vi "Crv_Info_Pan.vi"(8 "error in (no error)":errorcluster caption="entrée d'erreur (pas d'erreur)") -> (0 "error out":errorcluster caption="sortie d'erreur")   [LabVIEW 2019]
panel:
  out "EdPanelName":string="Scale & Offset"
  in  "Y Scale":dbl=60.0 min=0.1 step=0.1 format="%#.3f"
  in  "X Scale":dbl=60.0 min=0.1 step=0.1 format="%#.3f"
  in  "Y Offset":dbl caption="Offset" format="%.3f"
  in  "X Offset":dbl caption="Offset" format="%.3f"
  out "X Data Out":dbl[][](array[numeric])
  in  "XData":dbl[][](array[numeric])
  out "Y Data Out":dbl[][](array[numeric])
  in  "YData":dbl[][](array[numeric])
  in  "Apply_to":enum16{"X Data", "Y Data"}(ring) caption="Apply to:"
  in  "Quick Scale":dbl(slide) scale=0.0..6.0
  in  "Quick Offset":dbl(slide) scale=0.0..4.0
  in  "EditorProgQ":refnum<queue>
  in  "EditorProgQEvent":refnum<user-event>
  in  "Stop":bool
  in  "Offset":dbl format="%.3f"
  in  "Scale":dbl=60.0 format="%#.3f"
  out "Init Program":bool
  # "this MUST be present and labeled \"Stop\""
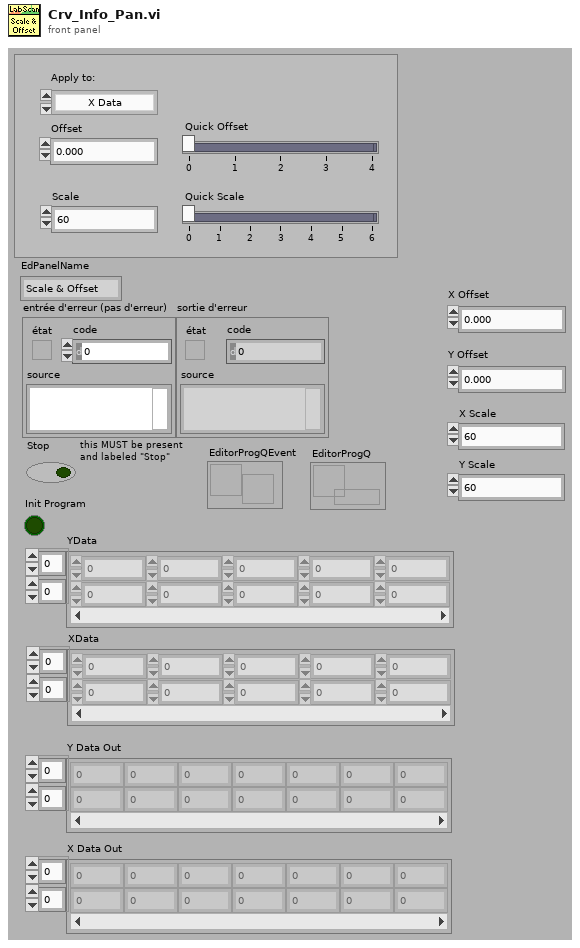
[diagram p1: front panel]
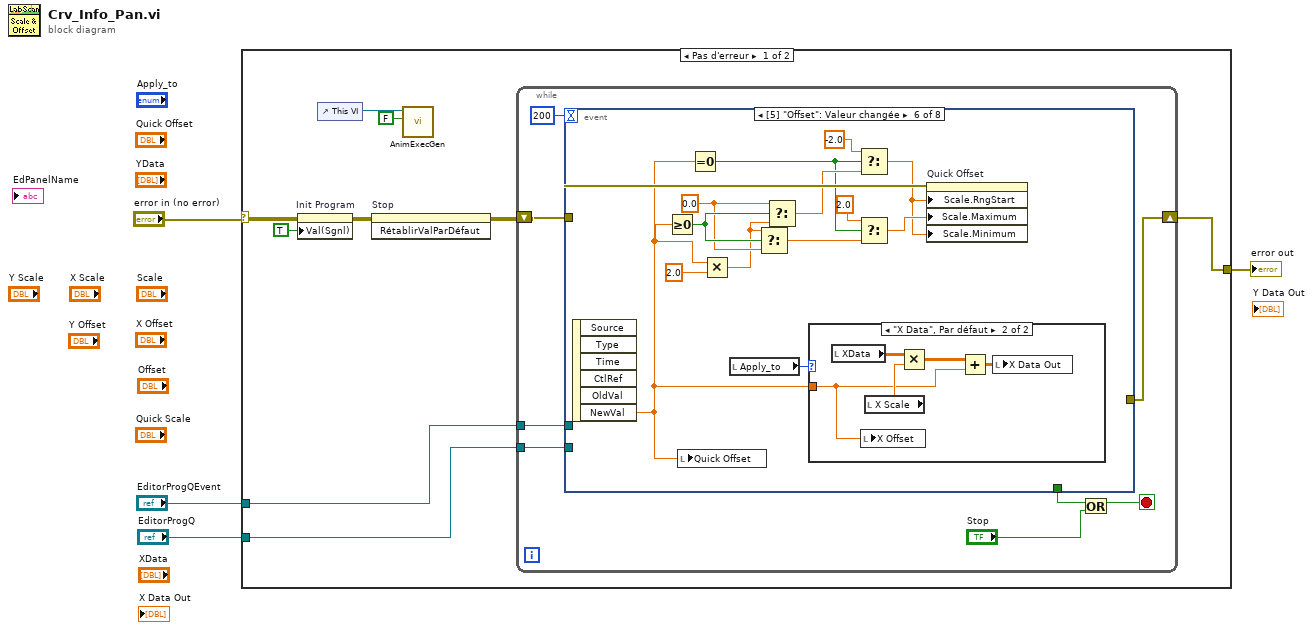
[diagram p0: block diagram]
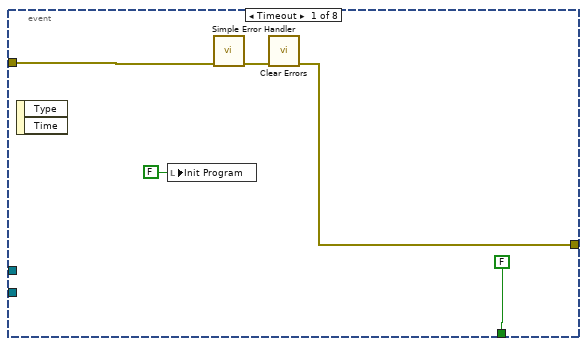
[diagram p2: hidden frame]
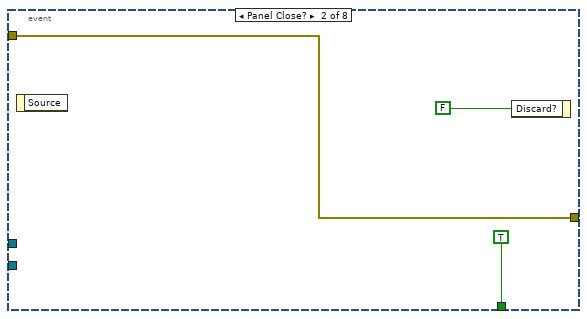
[diagram p3: hidden frame]
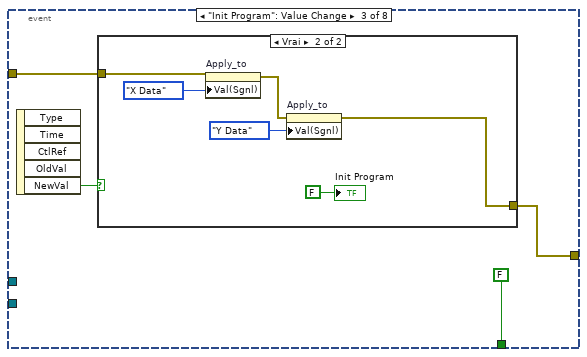
[diagram p4: hidden frame]
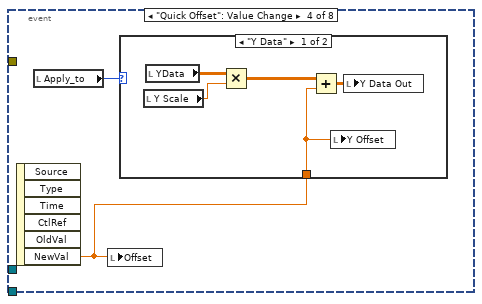
[diagram p6: hidden frame]
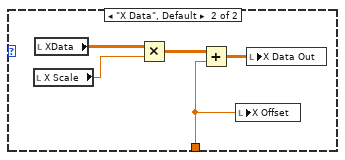
[diagram p7: hidden frame]
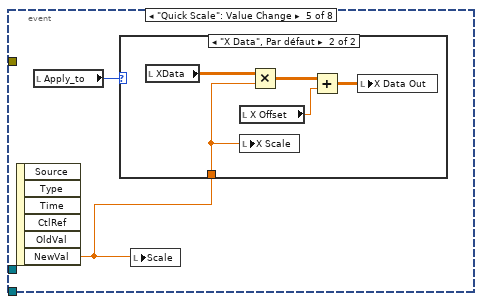
[diagram p8: hidden frame]
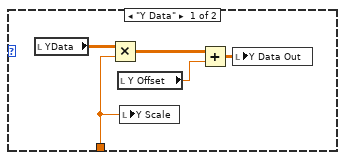
[diagram p9: hidden frame]
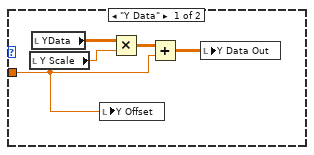
[diagram p10: hidden frame]
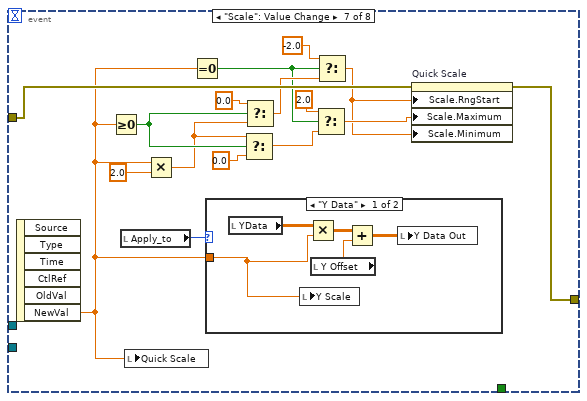
[diagram p11: hidden frame]
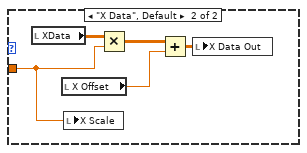
[diagram p12: hidden frame]
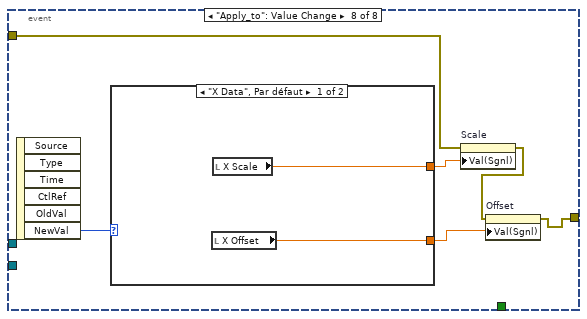
[diagram p13: hidden frame]
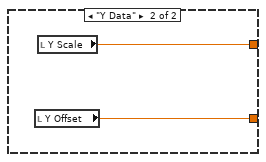
[diagram p14: hidden frame]
diagram:
  n1 = case shown="Pas d'erreur" "error in (no error)" {
    selector: "error in (no error)" -> [w11 w125]
    tunnel: [w13 w125] -> w3
    tunnel: "EditorProgQEvent" -> [w6 _]
    tunnel: "EditorProgQ" -> [w5 _]
    frame No Error {
      n2 = property on="Init Program" class="Bool (strict)"(error in=w11, "Val(Sgnl)"=TRUE ("Valeur (Signalisation)")) -> (error out=w10:errorcluster)  [unwired: 1 in, 1 out]
      n3 = control-ref of="This VI"() -> (w7:refnum<vi>)
      n4 = invoke on="Stop" class="Bool (strict)" method="RétablirValParDéfaut"(error in=w10) -> (error out=w9:errorcluster)  [unwired: 2 in, 2 out]
      n5 = call <userlib>:"AnimExecGen.vi"("Animer l'exécution ?"=FALSE, "ViRef"=w7) -> ()  [unwired: 9 in, 1 out]
      n6 = while {
        shift-right: [w19] -> w13
        shift-left: w9 -> [w20]
        tunnel: w6 -> [w15]
        tunnel: w5 -> [w14]
        stop <- w17 stop-if-true
        n7 = event shown="[5] \"Offset\": Valeur changée" {
          selector: _ -> [_ _ _ _ _ _ _ _]
          dyn-events: _ -> [_ _ _ _ _ _ _ _]
          timeout: 200 -> [_ _ _ _ _ _ _ _]
          tunnel: w20 -> [w25 w27 w32 _ _ w78 w104 w120]
          tunnel: [w23 w27 w31 _ _ _ w97 w115] -> w19
          tunnel: [FALSE TRUE FALSE _ _ _ _ _] -> w18
          tunnel: w15 -> [_ _ _ _ _ _ _ _]
          tunnel: w14 -> [_ _ _ _ _ _ _ _]
          event Timeout {
            n8 = event-data() -> ()  [unwired: 1 in, 2 out]
            n9 = local write "Init Program"(FALSE ("Init Program")) -> ()
            n10 = call <vilib>:"Simple Error Handler.vi"("error in (no error)"=w25) -> ("error out"=w24:errorcluster)  [unwired: 4 in, 4 out]
            n11 = call <vilib>:"Clear Errors.vi"("error in (no error)"=w24) -> ("error out"=w23:errorcluster)  [unwired: 5 in, 1 out]
          }
          event Panel Close? {
            n12 = event-data() -> ()  [unwired: 1 in, 1 out]
            n13 = event-data("Discard?"=FALSE ("Rejeter ?")) -> ()  [unwired: 1 in, 1 out]
          }
          event "Init Program": Value Change {
            n14 = event-data() -> ("NewVal"=w33:bool)  [unwired: 1 in, 4 out]
            n15 = case shown="Vrai" w33 {
              tunnel: w32 -> [w34 w37]
              tunnel: [w34 w39] -> w31
              frame False {
              }
              frame True {
                n16 = property on="Apply_to" class="Énum (strict)"(error in=w37, "Val(Sgnl)"=enum16{"X Data", "Y Data"}."X Data" ("Valeur (Signalisation)")) -> (error out=w36:errorcluster)  [unwired: 1 in, 1 out]
                n17 = property on="Apply_to" class="Énum (strict)"(error in=w36, "Val(Sgnl)"=enum16{"X Data", "Y Data"}."Y Data" ("Valeur (Signalisation)")) -> (error out=w39:errorcluster)  [unwired: 1 in, 1 out]
                "Init Program" <- FALSE
              }
            }
          }
          event "Quick Offset": Value Change {
            n18 = event-data() -> ("NewVal"=w42:dbl)  [unwired: 1 in, 5 out]
            n19 = local read "Apply_to"() -> (w41:enum16{"X Data", "Y Data"})
            n20 = local write "Offset"(w42) -> ()
            n21 = case shown="\"Y Data\"" w41 {
              tunnel: w42 -> [w46 w48]
              frame "Y Data" {
                n22 = local read "Y Scale"() -> (w43:dbl)
                n23 = local read "YData"() -> (w44:dbl[][])
                n24 = Multiply(x=w44, y=w43) -> (x*y=w45:dbl[][])
                n25 = Add(x=w45, y=w46) -> (x+y=w47:dbl[][])
                n26 = local write "Y Offset"(w46) -> ()
                n27 = local write "Y Data Out"(w47) -> ()
              }
              frame "X Data", Default {
                n28 = local read "X Scale"() -> (w49:dbl)
                n29 = local read "XData"() -> (w52:dbl[][])
                n30 = Multiply(x=w52, y=w49) -> (x*y=w50:dbl[][])
                n31 = Add(x=w50, y=w48) -> (x+y=w51:dbl[][])
                n32 = local write "X Offset"(w48) -> ()
                n33 = local write "X Data Out"(w51) -> ()
              }
            }
          }
          event "Quick Scale": Value Change {
            n34 = event-data() -> ("NewVal"=w54:dbl)  [unwired: 1 in, 5 out]
            n35 = local read "Apply_to"() -> (w53:enum16{"X Data", "Y Data"})
            n36 = case shown="\"X Data\", Par défaut" w53 {
              tunnel: w54 -> [w56 w61]
              frame "Y Data" {
                n37 = local read "YData"() -> (w57:dbl[][])
                n38 = Multiply(x=w57, y=w56) -> (x*y=w58:dbl[][])
                n39 = local read "Y Offset"() -> (w55:dbl)
                n40 = local write "Y Scale"(w56) -> ()
                n41 = Add(x=w58, y=w55) -> (x+y=w59:dbl[][])
                n42 = local write "Y Data Out"(w59) -> ()
              }
              frame "X Data", Default {
                n43 = local read "XData"() -> (w64:dbl[][])
                n44 = local read "X Offset"() -> (w60:dbl)
                n45 = local write "X Scale"(w61) -> ()
                n46 = Multiply(x=w64, y=w61) -> (x*y=w62:dbl[][])
                n47 = Add(x=w62, y=w60) -> (x+y=w63:dbl[][])
                n48 = local write "X Data Out"(w63) -> ()
              }
            }
            n49 = local write "Scale"(w54) -> ()
          }
          event "Offset": Value Change {
            w76 = 0.0 ("cas vrai")
            n50 = event-data() -> ("NewVal"=w73:dbl)  [unwired: 1 in, 5 out]
            n51 = Greater Or Equal To 0?(x=w73) -> (x >= 0?=w77:bool)
            n52 = local write "Quick Offset"(w73) -> ()
            n53 = Equal To 0?(x=w73) -> (x = 0?=w70:bool)
            n54 = Multiply(x=w73, y=2.0) -> (x*y=w66:dbl)
            n55 = local read "Apply_to"() -> (w75:enum16{"X Data", "Y Data"})
            n56 = Select(t=w66, s=w77, f=w76) -> (s? t:f=w69:dbl)
            n57 = Select(t=w76, s=w77, f=w66) -> (s? t:f=w72:dbl)
            n58 = case shown="\"X Data\", Par défaut" w75 {
              tunnel: w73 -> [w82 w84]
              frame "Y Data" {
                n59 = local read "Y Scale"() -> (w79:dbl)
                n60 = local read "YData"() -> (w80:dbl[][])
                n61 = local write "Y Offset"(w82) -> ()
                n62 = Multiply(x=w80, y=w79) -> (x*y=w81:dbl[][])
                n63 = Add(x=w81, y=w82) -> (x+y=w83:dbl[][])
                n64 = local write "Y Data Out"(w83) -> ()
              }
              frame "X Data", Default {
                n65 = local read "XData"() -> (w87:dbl[][])
                n66 = local write "X Offset"(w84) -> ()
                n67 = local read "X Scale"() -> (w85:dbl)
                n68 = Multiply(x=w87, y=w85) -> (x*y=w86:dbl[][])
                n69 = Add(x=w86, y=w84) -> (x+y=w88:dbl[][])
                n70 = local write "X Data Out"(w88) -> ()
              }
            }
            n71 = Select(t=-2.0 ("cas vrai"), s=w70, f=w72) -> (s? t:f=w65:dbl)
            n72 = Select(t=2.0 ("cas vrai"), s=w70, f=w69) -> (s? t:f=w68:dbl)
            n73 = property on="Quick Offset" class="Gliss (strict)"(error in=w78, "Scale.RngStart"=w65, "Scale.Maximum"=w68, "Scale.Minimum"=w65) -> ()  [unwired: 1 in, 2 out]
          }
          event "Scale": Value Change {
            n74 = event-data() -> ("NewVal"=w99:dbl)  [unwired: 1 in, 5 out]
            n75 = Greater Or Equal To 0?(x=w99) -> (x >= 0?=w103:bool)
            n76 = local read "Apply_to"() -> (w100:enum16{"X Data", "Y Data"})
            n77 = local write "Quick Scale"(w99) -> ()
            n78 = Multiply(x=w99, y=2.0) -> (x*y=w91:dbl)
            n79 = Equal To 0?(x=w99) -> (x = 0?=w96:bool)
            n80 = case shown="\"Y Data\"" w100 {
              tunnel: w99 -> [w106 w111]
              frame "Y Data" {
                n81 = local read "YData"() -> (w107:dbl[][])
                n82 = local write "Y Scale"(w106) -> ()
                n83 = Multiply(x=w107, y=w106) -> (x*y=w108:dbl[][])
                n84 = local read "Y Offset"() -> (w105:dbl)
                n85 = Add(x=w108, y=w105) -> (x+y=w109:dbl[][])
                n86 = local write "Y Data Out"(w109) -> ()
              }
              frame "X Data", Default {
                n87 = local read "XData"() -> (w113:dbl[][])
                n88 = local read "X Offset"() -> (w110:dbl)
                n89 = local write "X Scale"(w111) -> ()
                n90 = Multiply(x=w113, y=w111) -> (x*y=w112:dbl[][])
                n91 = Add(x=w112, y=w110) -> (x+y=w114:dbl[][])
                n92 = local write "X Data Out"(w114) -> ()
              }
            }
            n93 = Select(t=w91, s=w103, f=0.0 ("cas vrai")) -> (s? t:f=w95:dbl)
            n94 = Select(t=0.0 ("cas vrai"), s=w103, f=w91) -> (s? t:f=w98:dbl)
            n95 = Select(t=2.0 ("cas vrai"), s=w96, f=w95) -> (s? t:f=w94:dbl)
            n96 = Select(t=-2.0 ("cas vrai"), s=w96, f=w98) -> (s? t:f=w89:dbl)
            n97 = property on="Quick Scale" class="Gliss (strict)"(error in=w104, "Scale.RngStart"=w89, "Scale.Maximum"=w94, "Scale.Minimum"=w89) -> (error out=w97:errorcluster)  [unwired: 1 in, 1 out]
          }
          event "Apply_to": Value Change {
            n98 = event-data() -> ("NewVal"=w119:enum16{"X Data", "Y Data"})  [unwired: 1 in, 5 out]
            n99 = case shown="\"X Data\", Par défaut" w119 {
              tunnel: [w122 w124] -> w118
              tunnel: [w121 w123] -> w116
              frame "X Data", Default {
                n100 = local read "X Offset"() -> (w121:dbl)
                n101 = local read "X Scale"() -> (w122:dbl)
              }
              frame "Y Data" {
                n102 = local read "Y Offset"() -> (w123:dbl)
                n103 = local read "Y Scale"() -> (w124:dbl)
              }
            }
            n104 = property on="Scale" class="NumNb (strict)"(error in=w120, "Val(Sgnl)"=w118) -> (error out=w117:errorcluster)  [unwired: 1 in, 1 out]
            n105 = property on="Offset" class="NumNb (strict)"(error in=w117, "Val(Sgnl)"=w116) -> (error out=w115:errorcluster)  [unwired: 1 in, 1 out]
          }
        }
        n106 = Or(x=w18, y="Stop") -> (x .or. y?=w17:bool)
      }
    }
    frame Error {
    }
  }
  "error out" <- w3
